vi "example_02_upload.vi"() -> ()   [LabVIEW 2015, in "lv-dropbox.lvlib" / "v2.lvlib"]
uses:
  v2.lvlib
  public/advanced/upload-session.vi
  public/advanced/upload-file.vi
panel:
  in  "timeout_ms":i32=10000
  in  "chunk_size_bytes":i64=157286400
  in  "file_to_upload":path
  in  "path":string
  in  "file":string
  out "error":errorcluster
  in  "upload_selection":enum32{"Helper", "Session", "File"}(radio)
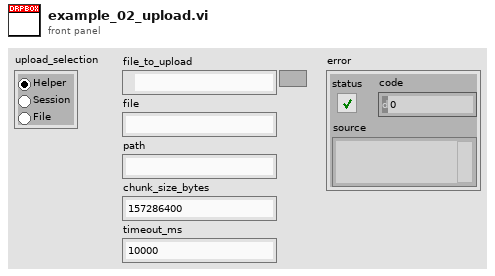
[diagram p1: front panel]
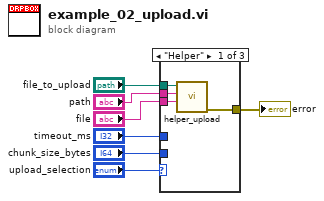
[diagram p0: block diagram]
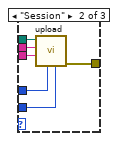
[diagram p2: hidden frame]
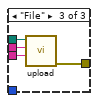
[diagram p3: hidden frame]
diagram:
  n1 = case shown="\"Helper\"" "upload_selection" {
    tunnel: [w11 w17 w21] -> w6
    tunnel: "file_to_upload" -> [w10 w16 w20]
    tunnel: "chunk_size_bytes" -> [_ w15 _]
    tunnel: "timeout_ms" -> [_ w14 _]
    tunnel: "path" -> [w9 w13 w19]
    tunnel: "file" -> [w8 w12 w18]
    frame "Helper" {
      n2 = call "helper_upload.vi"("file"=w8, "path"=w9, "filepath"=w10) -> ("error out"=w11:errorcluster)  [unwired: 8 in]
    }
    frame "Session" {
      n3 = call-poly "upload.vi"("chunk_size_bytes"=w15, "timeout_ms"=w14, "file"=w12, "path"=w13, "filepath"=w16) -> ("error out"=w17:errorcluster)  [unwired: 6 in]
    }
    frame "File" {
      n4 = call-poly "upload.vi"("file"=w18, "path"=w19, "filepath"=w20) -> ("error out"=w21:errorcluster)  [unwired: 8 in]
    }
  }
  "error" <- w6
